vi "Variance PtByPt.vi"(0 "x":dbl format="%0.2f", 1 "sample length":i32=100, 2 "initialize":bool) -> (3 "mean":dbl format="%0.2f", 4 "variance":dbl format="%0.2f", 5 "error":i32)   [LabVIEW 2017, in "NI_PtbyPt.lvlib"]
doc: "Computes the <B>variance</B> and <B>mean</B> of the set of input data points specified by <B>sample length</B>."
uses:
  <vilib>/ptbypt/NI_PtbyPt.lvlib
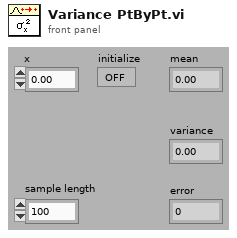
[diagram p1: front panel]
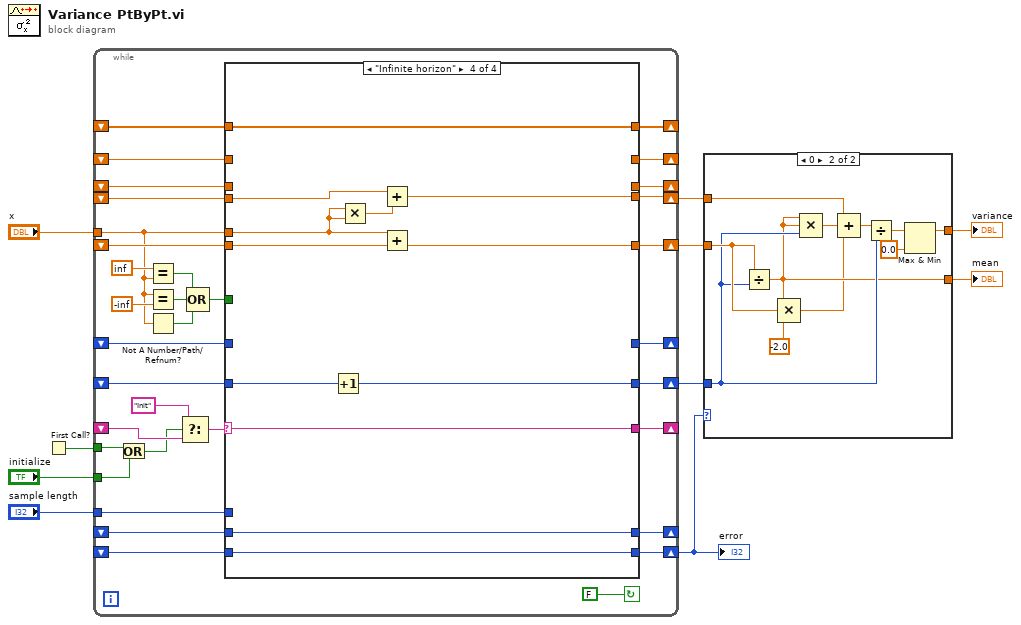
[diagram p0: block diagram]
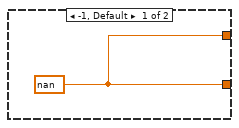
[diagram p2: hidden frame]
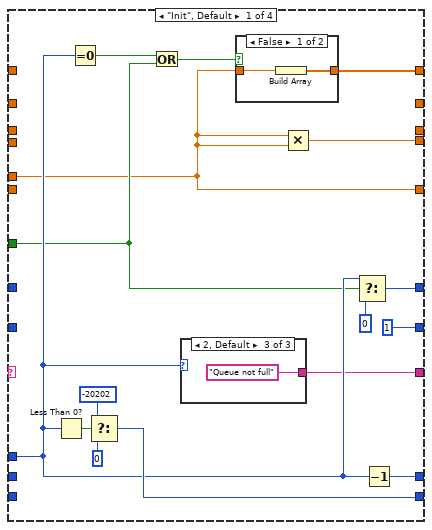
[diagram p3: hidden frame]
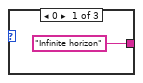
[diagram p5: hidden frame]
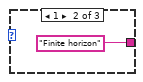
[diagram p6: hidden frame]
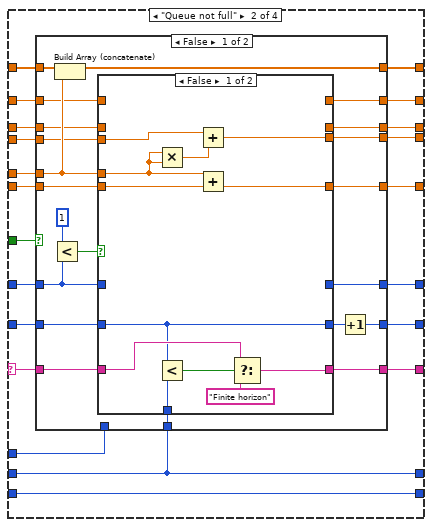
[diagram p7: hidden frame]
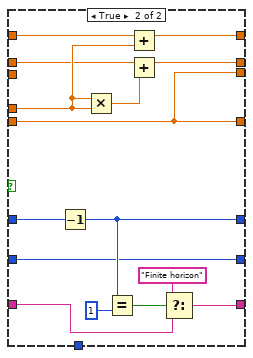
[diagram p8: hidden frame]
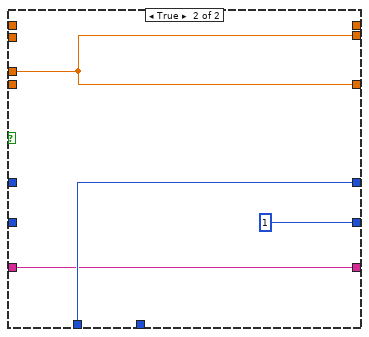
[diagram p9: hidden frame]
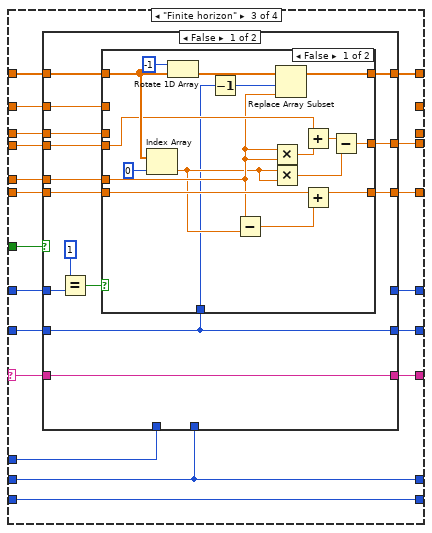
[diagram p10: hidden frame]
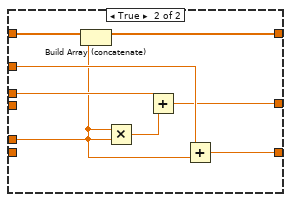
[diagram p11: hidden frame]
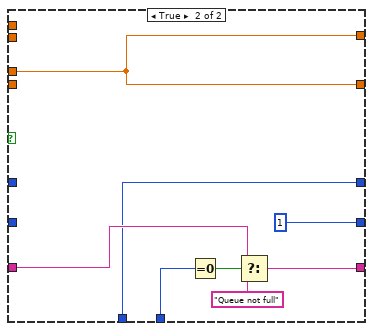
[diagram p12: hidden frame]
diagram:
  n1 = First Call?() -> (First Call?: T/F=w5:bool)
  n2 = while {
    tunnel: w5 -> [w29]
    shift-left: _ -> [w31]
    shift-right: [w32] -> _
    shift-left: _ -> [w33]
    shift-right: [w34] -> w9
    shift-left: _ -> [w36]
    shift-right: [w35] -> _
    shift-left: _ -> [w38]
    shift-right: [w39] -> w8
    shift-left: _ -> [w40]
    shift-right: [w41] -> w10
    shift-left: _ -> [w44]
    shift-right: [w37] -> _
    shift-right: [w21] -> _
    shift-left: _ -> [w20]
    shift-right: [w19] -> _
    shift-left: _ -> [w18]
    shift-right: [w17] -> _
    shift-left: _ -> [w16]
    shift-right: [w15] -> w4
    shift-left: _ -> [w14]
    tunnel: "x" -> [w13]
    tunnel: "sample length" -> [w12]
    tunnel: "initialize" -> [w11]
    stop <- FALSE continue-if-true
    n3 = Or(x=w29, y=w11) -> (x .or. y?=w28:bool)
    n4 = Equal?(x=inf, y=w13) -> (x = y?=w24:bool)
    n5 = Equal?(x=w13, y=-inf) -> (x = y?=w25:bool)
    n6 = Not A Number/Path/Refnum?(number/path/refnum=w13) -> (NaN/Path/Refnum?=w23:bool)
    n7 = Select(t="Init", s=w28, f=w44) -> (s? t:f=w42:string)
    n8 = Compound Arithmetic op=OR(w24, w25, w23) -> (w22:bool)
    n9 = case shown="\"Infinite horizon\"" w42 {
      selector: w42 -> [_ w82 w148 w213]
      tunnel: [w45 w84 w154 w215] -> w41
      tunnel: w40 -> [_ w78 w151 w216]
      tunnel: w13 -> [w45 w80 w150 w209]
      tunnel: [1 w75 w149 w205] -> w39
      tunnel: w38 -> [_ w83 w157 w214]
      tunnel: [w50 w81 w147 w213] -> w37
      tunnel: w36 -> [_ w86 w155 w212]
      tunnel: [w46 w85 w156 w212] -> w35
      tunnel: w12 -> [w51 w67 w141 _]
      tunnel: [w56 w79 w152 w208] -> w34
      tunnel: w33 -> [_ w77 w153 w211]
      tunnel: [w55 w76 w142 w207] -> w32
      tunnel: w31 -> [_ w76 w142 w207]
      tunnel: w22 -> [w48 w74 w146 _]
      tunnel: [w54 w68 w140 _] -> w21
      tunnel: w20 -> [_ w69 w145 _]
      tunnel: [_ w73 _ _] -> w19
      tunnel: w18 -> [_ w72 w144 _]
      tunnel: [_ w71 _ _] -> w17
      tunnel: w16 -> [_ w70 w143 _]
      tunnel: [w52 w66 w139 w206] -> w15
      tunnel: w14 -> [_ w66 w139 w206]
      frame "Init", Default {
        n10 = Less Than 0?(x=w51) -> (x < 0?=w57:bool)
        n11 = Equal To 0?(x=w51) -> (x = 0?=w49:bool)
        n12 = Select(t=-20202, s=w57, f=0) -> (s? t:f=w52:i32)
        n13 = Or(x=w49, y=w48) -> (x .or. y?=w47:bool)
        n14 = case shown="2, Default" w51 {
          tunnel: ["Infinite horizon" "Finite horizon" "Queue not full" ("f")] -> w50
          frame 0 {
          }
          frame 1 {
          }
          frame 2, Default {
          }
        }
        n15 = case shown="False" w47 {
          tunnel: [w62 _] -> w46
          tunnel: w45 -> [w61 _]
          frame False {
            n16 = Build Array(w61) -> (w62:dbl[])
          }
          frame True {
          }
        }
        n17 = Multiply(x=w45, y=w45) -> (x*y=w56:dbl)
        n18 = Select(t=w51, s=w48, f=0) -> (s? t:f=w54:i32)
        n19 = Decrement(x=w51) -> (x-1=w55:i32)
      }
      frame "Queue not full" {
        n20 = case shown="False" w74 {
          tunnel: w86 -> [w107 _]
          tunnel: [w106 _] -> w85
          tunnel: [w105 w138] -> w84
          tunnel: w83 -> [w104 _]
          tunnel: w82 -> [w103 w136]
          tunnel: [w102 w136] -> w81
          tunnel: w80 -> [w101 w138]
          tunnel: [w100 w138] -> w79
          tunnel: w78 -> [w99 _]
          tunnel: w77 -> [w98 _]
          tunnel: w76 -> [w97 _]
          tunnel: [w96 1] -> w75
          tunnel: [w94 _] -> w73
          tunnel: w72 -> [w93 _]
          tunnel: [w92 _] -> w71
          tunnel: w70 -> [w91 _]
          tunnel: w69 -> [w88 _]
          tunnel: [w90 w137] -> w68
          tunnel: w67 -> [_ w137]
          frame False {
            n21 = Less?(x=1, y=w88) -> (x < y?=w87:bool)
            n22 = Build Array (concatenate)(w107, w101) -> (w106:dbl[])
            n23 = case shown="False" w87 {
              tunnel: [w119 w128] -> w105
              tunnel: w104 -> [w108 w122]
              tunnel: w103 -> [w117 w121]
              tunnel: [w115 w120] -> w102
              tunnel: w101 -> [w114 w134]
              tunnel: [w113 w128] -> w100
              tunnel: w99 -> [w112 w128]
              tunnel: w98 -> [w111 _]
              tunnel: w97 -> [w109 _]
              tunnel: [w108 w122] -> w95
              tunnel: [_ w133] -> w94
              tunnel: w93 -> [_ w132]
              tunnel: [_ w130] -> w92
              tunnel: w91 -> [_ w129]
              tunnel: w88 -> [_ w124]
              tunnel: [_ w123] -> w90
              frame False {
                n24 = Multiply(x=w114, y=w114) -> (x*y=w110:dbl)
                n25 = Less?(x=w108, y=w109) -> (x < y?=w118:bool)
                n26 = Add(x=w111, y=w110) -> (x+y=w113:dbl)
                n27 = Add(x=w114, y=w112) -> (x+y=w119:dbl)
                n28 = Select(t=w117, s=w118, f="Finite horizon") -> (s? t:f=w115:string)
              }
              frame True {
                n29 = Decrement(x=w124) -> (x-1=w123:i32)
                n30 = Multiply(x=w134, y=w134) -> (x*y=w131:dbl)
                n31 = Equal?(x=w123, y=1) -> (x = y?=w127:bool)
                n32 = Add(x=w132, y=w134) -> (x+y=w133:dbl)
                n33 = Add(x=w129, y=w131) -> (x+y=w130:dbl)
                n34 = Select(t="Finite horizon" ("f"), s=w127, f=w121) -> (s? t:f=w120:string)
              }
            }
            n35 = Increment(x=w95) -> (x+1=w96:i32)
          }
          frame True {
          }
        }
      }
      frame "Finite horizon" {
        n36 = case shown="False" w146 {
          tunnel: w157 -> [w164 _]
          tunnel: [w171 _] -> w156
          tunnel: w155 -> [w170 _]
          tunnel: [w169 w197] -> w154
          tunnel: w153 -> [w168 _]
          tunnel: [w167 w197] -> w152
          tunnel: w151 -> [w166 _]
          tunnel: w150 -> [w165 w197]
          tunnel: [w164 1] -> w149
          tunnel: w148 -> [w163 w200]
          tunnel: [w163 w202] -> w147
          tunnel: w145 -> [w162 _]
          tunnel: w144 -> [w159 _]
          tunnel: w143 -> [w158 _]
          tunnel: w142 -> [_ w201]
          tunnel: w141 -> [_ w199]
          tunnel: [_ w199] -> w140
          frame False {
            n37 = Equal?(x=1, y=w162) -> (x = y?=w160:bool)
            n38 = case shown="False" w160 {
              tunnel: [w184 w191] -> w171
              tunnel: w170 -> [w183 w195]
              tunnel: [w182 w189] -> w169
              tunnel: w168 -> [w181 _]
              tunnel: [w177 w190] -> w167
              tunnel: w166 -> [w176 _]
              tunnel: w165 -> [w175 w192]
              tunnel: w164 -> [w172 _]
              tunnel: w159 -> [_ w194]
              tunnel: w158 -> [_ w193]
              frame False {
                n39 = Index Array(array=w183, index=0 ("Index")) -> (element=w174:dbl)
                n40 = Rotate 1D Array(1:w183, 2:i16 -1 ("n")) -> (0:w186:dbl[])
                n41 = Decrement(x=w172) -> (x-1=w185:i32)
                n42 = Subtract(x=w175, y=w174) -> (x-y=w173:dbl)
                n43 = Multiply(x=w175, y=w175) -> (x*y=w180:dbl)
                n44 = Multiply(x=w174, y=w174) -> (x*y=w178:dbl)
                n45 = Replace Array Subset(array=w186, new element=w175, index=w185) -> (w184:dbl[])
                n46 = Add(x=w181, y=w180) -> (x+y=w179:dbl)
                n47 = Add(x=w176, y=w173) -> (x+y=w182:dbl)
                n48 = Subtract(x=w179, y=w178) -> (x-y=w177:dbl)
              }
              frame True {
                n49 = Build Array (concatenate)(w195, w192) -> (w191:dbl[])
                n50 = Multiply(x=w192, y=w192) -> (x*y=w196:dbl)
                n51 = Add(x=w193, y=w196) -> (x+y=w190:dbl)
                n52 = Add(x=w194, y=w192) -> (x+y=w189:dbl)
              }
            }
          }
          frame True {
            n53 = Equal To 0?(x=w201) -> (x = 0?=w204:bool)
            n54 = Select(t=w200, s=w204, f="Queue not full") -> (s? t:f=w202:string)
          }
        }
      }
      frame "Infinite horizon" {
        n55 = Increment(x=w214) -> (x+1=w205:i32)
        n56 = Multiply(x=w209, y=w209) -> (x*y=w210:dbl)
        n57 = Add(x=w211, y=w210) -> (x+y=w208:dbl)
        n58 = Add(x=w209, y=w216) -> (x+y=w215:dbl)
      }
    }
  }
  "error" <- w4
  n59 = case shown="0" w4 {
    tunnel: w10 -> [_ w228]
    tunnel: w9 -> [_ w226]
    tunnel: w8 -> [_ w223]
    tunnel: [w217 w222] -> w7
    tunnel: [w217 w219] -> w6
    frame -1, Default {
      w217 = nan
    }
    frame 0 {
      n60 = Divide(x=w228, y=w223) -> (x/y=w222:dbl)
      n61 = Compound Arithmetic op=MULTIPLY(w222, w228, -2.0) -> (w221:dbl)
      n62 = Compound Arithmetic op=MULTIPLY(w222, w222, w223) -> (w225:dbl)
      n63 = Compound Arithmetic op=ADD(w226, w225, w221) -> (w224:dbl)
      n64 = Divide(x=w224, y=w223) -> (x/y=w220:dbl)
      n65 = Max & Min(x=w220, y=0.0) -> (max(x,y)=w219:dbl)  [unwired: 1 out]
    }
  }
  "variance" <- w6
  "mean" <- w7
